vi "NI 9775 1 Channel Continuous Mode (Host).vi"() -> ()   [LabVIEW 2021]
uses:
  <vilib>/userDefined/High Color/nirio_resource_hc.ctl
  <vilib>/LabVIEW Targets/FPGA/cRIO/shared/nicrio_ModuleControls/nicrio_cRIO-9775_ContinuousDataRates4ChansRing.ctl
  <vilib>/FPGAPlugInAG/cRIO-9053/niLvFpga_Open_cRIO-9053.vi
  <vilib>/rvi/interface/common/dynamic/niFpgaDynamicAddResources.vi
  <vilib>/FPGAPlugInAG/Dynamic/niLvFpga_Reset_Dynamic.vi
  <vilib>/Utility/error.llb/Error Cluster From Error Code.vi
  <vilib>/rvi/errors/niLvFpgaAdjustHostInterfaceError.vi
  <vilib>/FPGAPlugInAG/Dynamic/niLvFpga_Run_Dynamic.vi
  <vilib>/FPGAPlugInAG/Dynamic/niLvFpga_Close_Dynamic.vi
  <vilib>/rvi/interface/nirviOpenFPGA/nirviOpenFPGA.xnode
  FPGA Bitfiles/ni9775crio9053_FPGATarget2_NI97751ChannelCo_SIuNrVEWdDE.lvbitx
  NI 9775  1 Channel Continuous Mode (FPGA).vi
  <vilib>/rvi/interface/nirviMethod/nirviMethod.xnode
  <vilib>/rvi/interface/nirviReadWriteControl/nirviReadWriteControl.xnode
  <vilib>/rvi/interface/nirviCloseFPGA/nirviCloseFPGA.xnode
  <vilib>/rvi/interface/Simulation/niFpgaSimulationCallBeginRW.vi
  <vilib>/FPGAPlugInAG/Dynamic/niLvFpga_ReadFifo_Dynamic.vi
  <vilib>/rvi/errors/niLvFpgaMergeErrorWithErrorCode.vi
  NiFpgaLv.dll
panel:
  in  "Continuous Data Rate":T1=20 items=["1.000 MS/s (NI 9775)"=20, "833.333 KS/s (NI 9775)"=24, "714.286 KS/s (NI 9775)"=28, "625.000 KS/s (NI 9775)"=32, "555.556 KS/s (NI 9775)"=36, "500.000 KS/s (NI 9775)"=40, "454.545 KS/s (NI 9775)"=44, "416.667 KS/s (NI 9775)"=48, "384.615 KS/s (NI 9775)"=52, "357.143 KS/s (NI 9775)"=56, "333.333 KS/s (NI 9775)"=60, "312.500 KS/s (NI 9775)"=64, "294.118 KS/s (NI 9775)"=68, "277.778 KS/s (NI 9775)"=72, "263.158 KS/s (NI 9775)"=76, "250.000 KS/s (NI 9775)"=80, "238.095 KS/s (NI 9775)"=84, "227.273 KS/s (NI 9775)"=88, "217.391 KS/s (NI 9775)"=92, "208.333 KS/s (NI 9775)"=96, "200.000 KS/s (NI 9775)"=100, "192.308 KS/s (NI 9775)"=104, "185.185 KS/s (NI 9775)"=108, "178.571 KS/s (NI 9775)"=112, "172.414 KS/s (NI 9775)"=116, "166.667 KS/s (NI 9775)"=120, "161.290 KS/s (NI 9775)"=124, "156.250 KS/s (NI 9775)"=128, "151.515 KS/s (NI 9775)"=132, "147.059 KS/s (NI 9775)"=136, "142.857 KS/s (NI 9775)"=140, "138.889 KS/s (NI 9775)"=144, "135.135 KS/s (NI 9775)"=148, "131.579 KS/s (NI 9775)"=152, "128.205 KS/s (NI 9775)"=156, "125.000 KS/s (NI 9775)"=160, "121.951 KS/s (NI 9775)"=164, "119.048 KS/s (NI 9775)"=168, "116.279 KS/s (NI 9775)"=172, "113.636 KS/s (NI 9775)"=176, "111.111 KS/s (NI 9775)"=180, "108.696 KS/s (NI 9775)"=184, "106.383 KS/s (NI 9775)"=188, "104.167 KS/s (NI 9775)"=192, "102.041 KS/s (NI 9775)"=196, "100.000 KS/s (NI 9775)"=200, "50.000 KS/s (NI 9775)"=400, "33.333 KS/s (NI 9775)"=600, "25.000 KS/s (NI 9775)"=800, "20.000 KS/s (NI 9775)"=1000, "16.667 KS/s (NI 9775)"=1200, "14.286 KS/s (NI 9775)"=1400, "12.500 KS/s (NI 9775)"=1600, "11.111 KS/s (NI 9775)"=1800, "10.000 KS/s (NI 9775)"=2000, "9.091 KS/s (NI 9775)"=2200, "8.333 KS/s (NI 9775)"=2400, "7.692 KS/s (NI 9775)"=2600, "7.143 KS/s (NI 9775)"=2800, "6.667 KS/s (NI 9775)"=3000, "6.250 KS/s (NI 9775)"=3200, "5.882 KS/s (NI 9775)"=3400, "5.556 KS/s (NI 9775)"=3600, "5.000 KS/s (NI 9775)"=4000, "4.762 KS/s (NI 9775)"=4200, "4.545 KS/s (NI 9775)"=4400, "4.348 KS/s (NI 9775)"=4600, "4.167 KS/s (NI 9775)"=4800, "4.000 KS/s (NI 9775)"=5000, "3.846 KS/s (NI 9775)"=5200, "3.571 KS/s (NI 9775)"=5600, "3.333 KS/s (NI 9775)"=6000, "3.125 KS/s (NI 9775)"=6400, "2.941 KS/s (NI 9775)"=6800, "2.778 KS/s (NI 9775)"=7200, "2.632 KS/s (NI 9775)"=7600, "2.500 KS/s (NI 9775)"=8000, "2.381 KS/s (NI 9775)"=8400, "2.273 KS/s (NI 9775)"=8800, "2.174 KS/s (NI 9775)"=9200, "2.083 KS/s (NI 9775)"=9600, "2.000 KS/s (NI 9775)"=10000, "1.923 KS/s (NI 9775)"=10400, "1.852 KS/s (NI 9775)"=10800, "1.786 KS/s (NI 9775)"=11200, "1.724 KS/s (NI 9775)"=11600, "1.667 KS/s (NI 9775)"=12000, "1.613 KS/s (NI 9775)"=12400, "1.563 KS/s (NI 9775)"=12800, "1.515 KS/s (NI 9775)"=13200, "1.471 KS/s (NI 9775)"=13600, "1.429 KS/s (NI 9775)"=14000, "1.389 KS/s (NI 9775)"=14400, "1.351 KS/s (NI 9775)"=14800, "1.316 KS/s (NI 9775)"=15200, "1.282 KS/s (NI 9775)"=15600, "1.250 KS/s (NI 9775)"=16000, "1.220 KS/s (NI 9775)"=16400, "1.190 KS/s (NI 9775)"=16800, "1.163 KS/s (NI 9775)"=17200, "1.136 KS/s (NI 9775)"=17600, "1.111 KS/s (NI 9775)"=18000, "1.087 KS/s (NI 9775)"=18400, "1.064 KS/s (NI 9775)"=18800, "1.042 KS/s (NI 9775)"=19200, "1.020 KS/s (NI 9775)"=19600, "1.000 KS/s (NI 9775)"=20000, "0.980 KS/s (NI 9775)"=20400, "0.962 KS/s (NI 9775)"=20800, "0.943 KS/s (NI 9775)"=21200, "0.926 KS/s (NI 9775)"=21600, "0.909 KS/s (NI 9775)"=22000, "0.893 KS/s (NI 9775)"=22400, "0.877 KS/s (NI 9775)"=22800, "0.862 KS/s (NI 9775)"=23200, "0.847 KS/s (NI 9775)"=23600, "0.833 KS/s (NI 9775)"=24000, "0.820 KS/s (NI 9775)"=24400, "0.806 KS/s (NI 9775)"=24800, "0.794 KS/s (NI 9775)"=25200, "0.781 KS/s (NI 9775)"=25600, "0.694 KS/s (NI 9775)"=28800, "0.625 KS/s (NI 9775)"=32000, "0.568 KS/s (NI 9775)"=35200, "0.521 KS/s (NI 9775)"=38400, "0.446 KS/s (NI 9775)"=44800, "0.391 KS/s (NI 9775)"=51200, "0.347 KS/s (NI 9775)"=57600, "0.313 KS/s (NI 9775)"=64000]
  in  "Timing Mode":enum8{"High Speed", "High Resolution"}(ring)
  in  "Enable Low Pass Filter CH0":bool
  out "Host error out":errorcluster
  out "FPGA error out":errorcluster
  in  "stop":bool
  out "Waveform Graph":waveform(dbl)(graph)
  out "Elements Remaining":u32
  out "Data FIFO Full":bool
  in  "Host Loop update rate (ms)":u32=100
  in  "RIO Device":T2="RIO0"
  # "Overview: Demonstrates how to continuously acquire data from the NI 9775\nRequirements: LabVIEW Full Development System, LV FPGA, and NI RIO\nInstructions: \n1. Run the VI."
  # "FPGA Input Parameters"
  # "Timing Parameters"
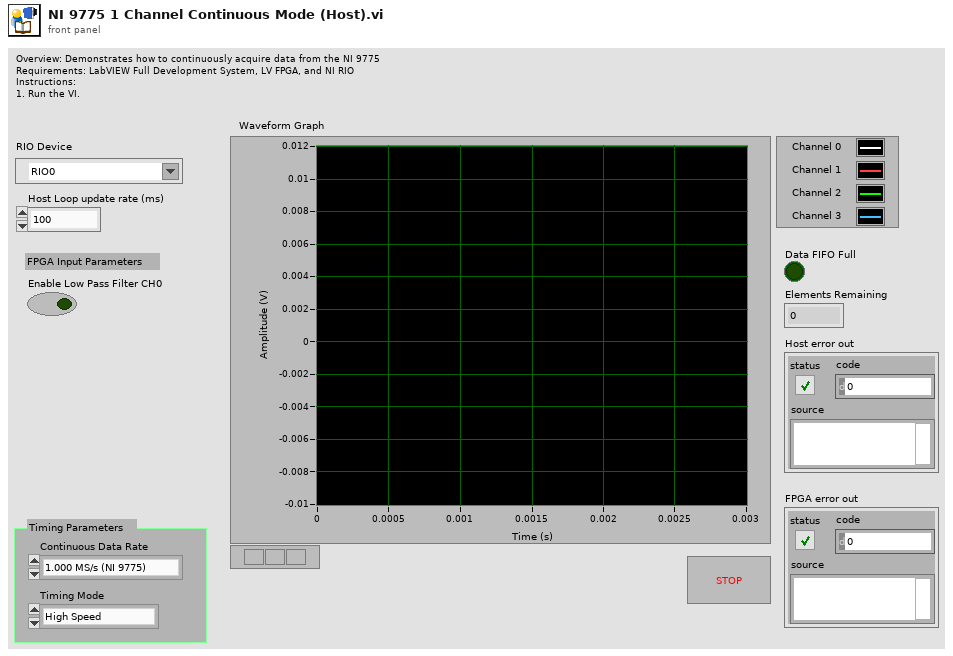
[diagram p1: front panel]
types:
  T1 = typedef "nicrio_cRIO-9775_ContinuousDataRates4ChansRing.ctl" = u16
  T2 = typedef "nirio_resource_hc.ctl" = tag
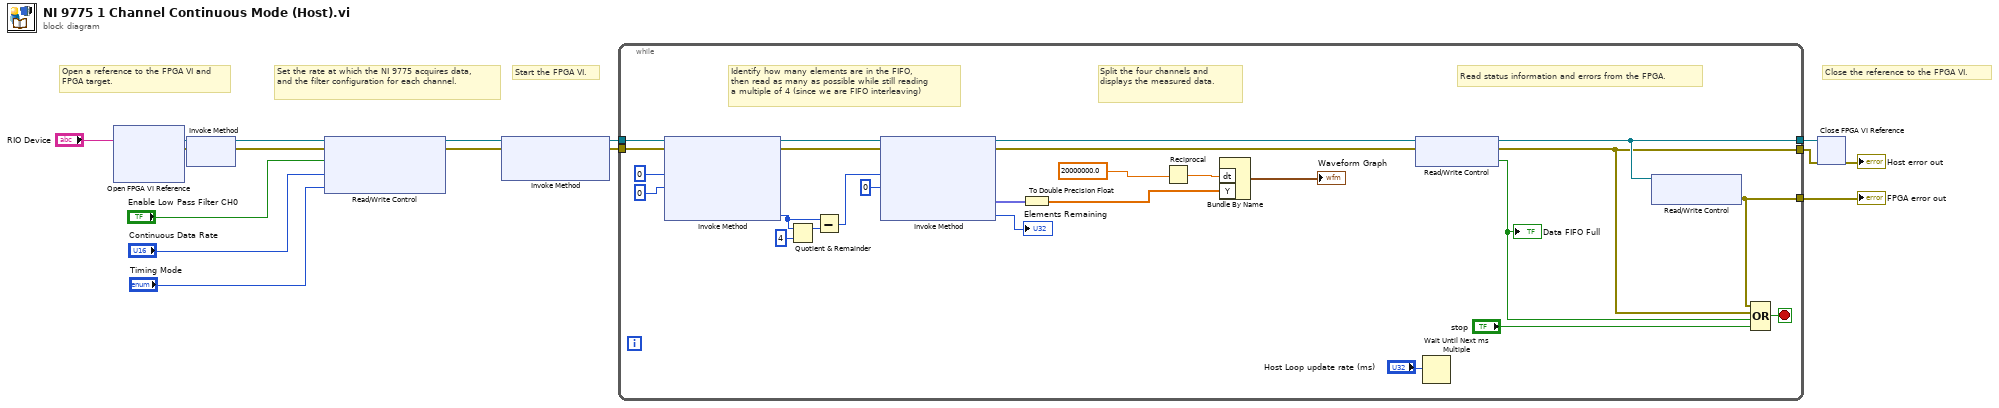
[diagram p0: block diagram]
diagram:
  # "Close the reference to the FPGA VI."
  # "Start the FPGA VI."
  # "Set the rate at which the NI 9775 acquires data, and the filter configuration for each channel."
  # "Open a reference to the FPGA VI and FPGA target."
  n1 = xnode "Open FPGA VI Reference"("resource name"="RIO Device") -> ("FPGA VI Reference Out"=w5:refnum<k20>, "error out"=w4:errorcluster)  [unwired: 1 in]
  n2 = xnode "Invoke Method"("FPGA VI Reference In"=w5, "error in"=w4) -> ("FPGA VI Reference Out"=w8:refnum<k20>, "error out"=w9:errorcluster)
  n3 = xnode "Read/Write Control"("FPGA VI Reference In"=w8, "error in"=w9, "Enable Analog Filter"="Enable Low Pass Filter CH0", "Continuous Data Rate"="Continuous Data Rate", "Timing Mode"="Timing Mode") -> ("FPGA VI Reference Out"=w12:refnum<k20>, "error out"=w13:errorcluster)
  n4 = xnode "Invoke Method"("FPGA VI Reference In"=w12, "error in"=w13) -> ("FPGA VI Reference Out"=w15:refnum<k20>, "error out"=w16:errorcluster)  [unwired: 1 in]
  n5 = while {
    tunnel: w16 -> [w24]
    tunnel: w15 -> [w25]
    tunnel: [w33] -> w14
    tunnel: [w32] -> w11
    tunnel: [w31] -> w7
    stop <- w42 stop-if-true
    # "Split the four channels and displays the measured data."
    # "Read status information and errors from the FPGA."
    # "Identify how many elements are in the FIFO, \nthen read as many as possible while still reading\na multiple of 4 (since we are FIFO interleaving)"
    n6 = xnode "Invoke Method"("FPGA VI Reference In"=w25, "error in"=w24, "Number of Elements"=u32 0, "Timeout (ms)"=0) -> ("FPGA VI Reference Out"=w23:refnum<k20>, "error out"=w22:errorcluster, "Elements Remaining"=w26:u32)  [unwired: 1 out]
    n7 = Quotient & Remainder(x=w26, y=u32 4) -> (x-y*floor(x/y)=w27:u32)  [unwired: 1 out]
    n8 = Subtract(x=w26, y=w27) -> (x-y=w21:u32)
    n9 = xnode "Invoke Method"("FPGA VI Reference In"=w23, "error in"=w22, "Number of Elements"=w21, "Timeout (ms)"=0 ("Timeout")) -> ("FPGA VI Reference Out"=w39:refnum<k20>, "error out"=w38:errorcluster, "Data"=w34:fxp<+/-,17,5>[], "Elements Remaining"=→"Elements Remaining":u32)
    n10 = To Double Precision Float(number=w34) -> (double precision float=w17:dbl[])
    n11 = Reciprocal(x=20000000.0) -> (1/x=w36:dbl)
    n12 = Bundle By Name("dt"=w36, "Y"=w17) -> (→"Waveform Graph":waveform(dbl))  [unwired: 1 out]
    n13 = xnode "Read/Write Control"("FPGA VI Reference In"=w39, "error in"=w38) -> ("FPGA VI Reference Out"=w33:refnum<k20>, "error out"=w32:errorcluster, "Data FIFO Full"=w41:bool)
    "Data FIFO Full" <- w41
    n14 = Wait Until Next ms Multiple(millisecond multiple="Host Loop update rate (ms)") -> ()  [unwired: 1 out]
    n15 = xnode "Read/Write Control"("FPGA VI Reference In"=w33) -> ("FPGA Error Out"=w31:errorcluster)  [unwired: 1 in, 2 out]
    n16 = Compound Arithmetic op=OR(w31, w32, w41, "stop") -> (w42:bool)
  }
  "FPGA error out" <- w7
  n17 = xnode "Close FPGA VI Reference"("FPGA VI Reference In"=w14, "error in"=w11) -> ("error out"=→"Host error out":errorcluster)
